vi "Agilent SNA Measure.vi"(5 "Miscellaneous Parameters":T1, 7 "Agilent SNA & SWP":T6, 8 "error in (no error)":errorcluster, 9 "SP Stimulus":T2={"Use Instrument Settings"=FALSE, "Blank Frequencies"=FALSE, "Sweep Type"=enum."Linear", "Sweep"={"Fstart"=500.0, "Fstop"=1500.0, "Units"=enum."MHz", "Points"=201}, "Power (dBm)"=999.0, "IFBW (Hz)"=-1.0, "Sweep Time (s)"=-1.0, "Calibration"={"State"=FALSE, "String"=""}} {"Sweep Time (s)" format="%.3g"}, 10 "Parameters to Measure":T7[](array[typedef]) {"Channel" min=1 max=99 step=1; "Parameter"."Stimulus Port" min=1 step=1; "Parameter"."Response Port" min=1 step=1}, 11 "VISA Resource Names":T5) -> (0 "error out":errorcluster, 1 "S Parameters":cluster{"f0":dbl, "df":dbl, cdb[][]}, 2 "Parameters to Measure":T7[](array[typedef]) {"Channel" min=1 max=99 step=1; "Parameter"."Stimulus Port" min=1 step=1; "Parameter"."Response Port" min=1 step=1}, 3 "dup VISA Resource Names":T5)   [LabVIEW 2011]
uses:
  tests/S Parameter/TypeDefs/SP Parameter to Measure.ctl
  tests/S Parameter/TypeDefs/SP Parameter.ctl
  tests/S Parameter/TypeDefs/SP Calibration State.ctl
  tests/S Parameter/TypeDefs/SP Measurement Format.ctl
  TypeDefs/Agilent SNA VISA.ctl
  TypeDefs/Agilent SNA Instrument Info.ctl
  tests/S Parameter/TypeDefs/SP Stimulus Parameters.ctl
  tests/S Parameter/TypeDefs/SP Frequency Units.ctl
  tests/S Parameter/TypeDefs/SP Miscellaneous Parameters.ctl
  TypeDefs/Agilent SNA Message Mode.ctl
  TypeDefs/Agilent SNA Measurement.ctl
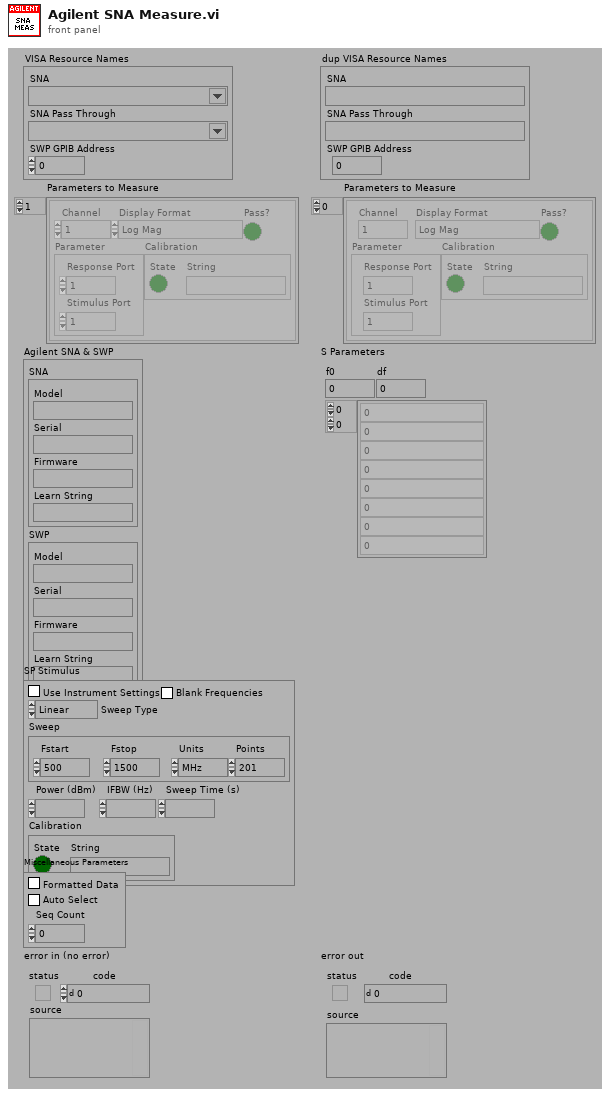
[diagram p1: front panel]
types:
  T1 = typedef "SP Miscellaneous Parameters.ctl" = cluster{"Formatted Data":bool, "Auto Select":bool, "Seq Count":u32}
  T2 = typedef "SP Stimulus Parameters.ctl" = cluster{"Use Instrument Settings":bool, "Blank Frequencies":bool, "Sweep Type":enum32{"Linear", "Logarithmic", "List", "Power", "CW"}, "Sweep":cluster{"Fstart":dbl, "Fstop":dbl, "Units":T3, "Points":i32}, "Power (dBm)":dbl, "IFBW (Hz)":dbl, "Sweep Time (s)":dbl, "Calibration":T4}
  T3 = typedef "SP Frequency Units.ctl" = enum16{"Hz", "kHz", "MHz", "GHz", "Points"}
  T4 = typedef "SP Calibration State.ctl" = cluster{"State":bool, "String":string}
  T5 = typedef "Agilent SNA VISA.ctl" = cluster{"SNA":refnum<visa-resource-name>, "SNA Pass Through":refnum<visa-resource-name>, "SWP GPIB Address":i32}
  T6 = typedef "Agilent SNA Instrument Info.ctl" = cluster{"SNA":cluster{"Model":string, "Serial":string, "Firmware":string, "Learn String":string}, "SWP":cluster{"Model":string, "Serial":string, "Firmware":string, "Learn String":string}}
  T7 = typedef "SP Parameter to Measure.ctl" = cluster{"Channel":i8, "Parameter":T8, "Calibration":T4, "Display Format":T9, "Pass?":bool}
  T8 = typedef "SP Parameter.ctl" = cluster{"Stimulus Port":i8, "Response Port":i8}
  T9 = typedef "SP Measurement Format.ctl" = enum32{"Log Mag", "Phase", "Delay", "Smith (R+jX)", "Polar (Re/Im)", "Linear Mag", "SWR", "Real", "Imaginary", "Smith (Lin/Phase)", "Smith (Log/Phase)", "Smith (Real/Imag)", "Smith (G+jB)", "Polar (Lin/Phase)", "Polar (Log/Phase)", "Expanded Phase", "Positive Phase", "Inverted Smith", "Unwrapped Phase", "Power Out", "Power In", "Linear Mag/Phase", "Log Mag/Phase", "Real/Imaginary"}
  T10 = typedef "Agilent SNA Message Mode.ctl" = enum16{"On", "Off"}
  T11 = typedef "Agilent SNA Model.ctl" = enum16{"Not Supported", "8757X"}
  T12 = typedef "Agilent SNA Measurement.ctl" = enum32{"SXX", "A", "B", "C", "R", "A/B", "A/C", "A/R", "B/A", "B/C", "B/R", "C/A", "C/B", "C/R", "R/A", "R/B", "R/C", "Analog In - Aux In"}
  T13 = typedef "Agilent SNA Measurements.ctl" = cluster{"Channel":i8, "Traces":cluster{"Trace":i8, "Parameter":T8}[]}
  T14 = typedef "Agilent SNA Trigger Mode.ctl" = enum16{"Continuous", "Hold", "Single"}
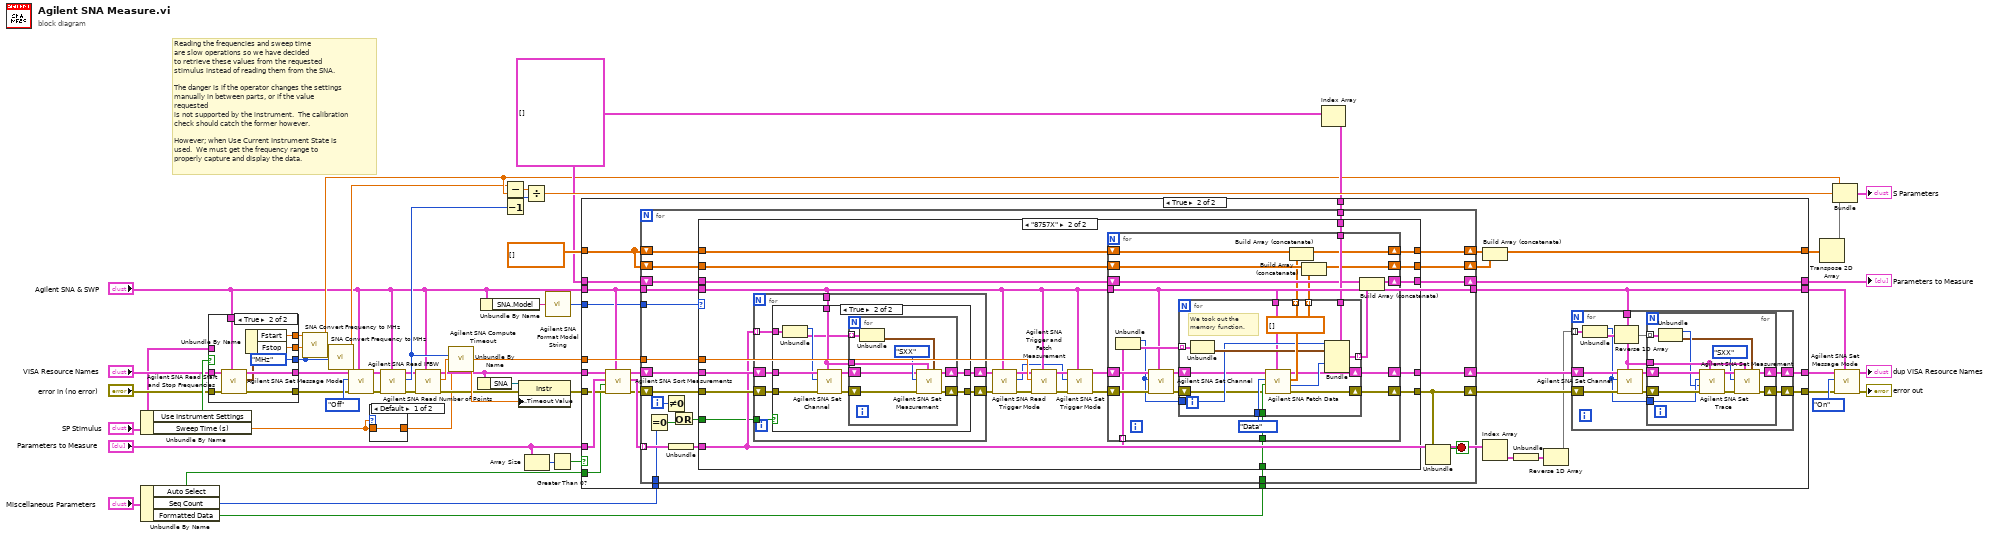
[diagram p0: block diagram]
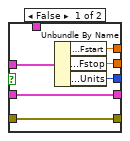
[diagram p2: hidden frame]
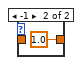
[diagram p3: hidden frame]
diagram:
  w33 = T7[] [] ("Parameters to Measure")
  # "Reading the frequencies and sweep time\nare slow operations so we have decided\nto retrieve these values from the requested\nstimulus instead of reading them from the SNA.\n\nThe danger is if the operator changes the settings\nmanually in between parts, or if the value requested\nis not supported by the instrument.  The calibration\ncheck should catch the former however.\n\nHowever; when Use Current Instrument State is\nused.  We must get the frequency range to\nproperly capture and display the data."
  n1 = Unbundle By Name("SP Stimulus") -> ("Use Instrument Settings"=w10:bool, "Sweep Time (s)"=w26:dbl)
  n2 = Unbundle By Name("Miscellaneous Parameters") -> ("Auto Select"=w34:bool, "Seq Count"=w28:u32, "Formatted Data"=w29:bool)
  n3 = case shown="True" w10 {
    tunnel: "VISA Resource Names" -> [w56 w63]
    tunnel: "error in (no error)" -> [w57 w66]
    tunnel: [w57 w65] -> w7
    tunnel: [w56 w64] -> w6
    tunnel: "Agilent SNA & SWP" -> [_ w62]
    tunnel: "SP Stimulus" -> [w55 _]
    tunnel: [w54 w60] -> w3
    tunnel: [w53 w59] -> w2
    tunnel: [w52 SP_Frequency_Units."MHz" ("Units")] -> w1
    frame False {
      n4 = Unbundle By Name(w55) -> ("Sweep.Fstart"=w54:dbl, "Sweep.Fstop"=w53:dbl, "Sweep.Units"=w52:T3)
    }
    frame True {
      n5 = call "Agilent SNA Read Start and Stop Frequencies.vi"("Agilent SNA & SWP"=w62, "error in (no error)"=w66, "VISA Resource Names"=w63) -> ("error out"=w65:errorcluster, "Start/Stop Freqs, MHz"=w61:cluster{"Fstart":dbl, "Fstop":dbl}, "dup VISA Resource Names"=w64:T5)  [unwired: 2 in, 4 out]
      n6 = Unbundle By Name(w61) -> ("Fstart"=w60:dbl, "Fstop"=w59:dbl)
    }
  }
  n7 = call "SNA Convert Frequency to MHz.vi"("Units"=w1, "Frequency"=w3) -> ("Converted Frequency"=w21:dbl)  [unwired: 9 out]
  n8 = call "SNA Convert Frequency to MHz.vi"("Units"=w1, "Frequency"=w2) -> ("Converted Frequency"=w20:dbl)  [unwired: 9 out]
  n9 = call "Agilent SNA Set Message Mode.vi"("Agilent SNA & SWP"="Agilent SNA & SWP", "error in (no error)"=w7, "Message Mode"=Agilent_SNA_Message_Mode."Off", "VISA Resource Names"=w6) -> ("error out"=w16:errorcluster, "dup VISA Resource Names"=w17:T5)  [unwired: 6 out]
  n10 = case shown="Default" w26 {
    tunnel: w26 -> [w67 _]
    tunnel: [w67 1.0 ("Sweep Time (s)")] -> w22
    frame Default {
    }
    frame -1 {
    }
  }
  n11 = call "Agilent SNA Read Number of Points.vi"("Agilent SNA & SWP"="Agilent SNA & SWP", "error in (no error)"=w16, "VISA Resource Names"=w17) -> ("error out"=w38:errorcluster, "Number Points"=w40:i32, "dup VISA Resource Names"=w39:T5)  [unwired: 1 in, 5 out]
  n12 = call "Agilent SNA Read IFBW.vi"("Agilent SNA & SWP"="Agilent SNA & SWP", "error in (no error)"=w38, "VISA Resource Names"=w39) -> ("error out"=w23:errorcluster, "IFBW, Hz"=w25:dbl, "dup VISA Resource Name"=w24:T5)  [unwired: 1 in, 5 out]
  n13 = call "Agilent SNA Compute Timeout.vi"("Points"=w40, "IFBW (Hz)"=w25, "Sweep Time (s)"=w22) -> ("Timeout (ms)"=w41:dbl)  [unwired: 1 in, 11 out]
  n14 = Unbundle By Name(w24) -> ("SNA"=w27:refnum<visa-resource-name>)
  n15 = Unbundle By Name("Agilent SNA & SWP") -> ("SNA.Model"=w31:string)
  n16 = Subtract(x=w20, y=w21) -> (x-y=w50:dbl)
  n17 = Decrement(x=w40) -> (x-1=w49:i32)
  n18 = property class="Instr"(reference=w27, error in=w23, "General Settings:Timeout Value"=w41) -> (error out=w43:errorcluster)  [unwired: 1 out]
  n19 = Divide(x=w50, y=w49) -> (x/y=w47:dbl)
  n20 = Array Size(array="Parameters to Measure") -> (size(s)=w45:i32)
  n21 = call "Agilent SNA Format Model String.vi"("Model String"=w31) -> ("Model"=w30:T11)
  n22 = Greater Than 0?(x=w45) -> (x > 0?=w44:bool)
  n23 = Index Array(array=w33) -> (element=w32:T7)  [unwired: 1 in]
  n24 = case shown="True" w44 {
    tunnel: [w73 w95] -> w13
    tunnel: w24 -> [w71 w81]
    tunnel: "Parameters to Measure" -> [_ w100]
    tunnel: [w72 w88] -> w51
    tunnel: "Agilent SNA & SWP" -> [w69 w79]
    tunnel: w43 -> [w73 w84]
    tunnel: cdb[][] [] -> [w72 w91]
    tunnel: [w71 w94] -> w12
    tunnel: w41 -> [_ w92]
    tunnel: w29 -> [_ w87]
    tunnel: [w70 w86] -> w36
    tunnel: w33 -> [w70 w85]
    tunnel: w34 -> [_ w80]
    tunnel: w32 -> [_ w78]
    tunnel: w30 -> [_ w76]
    tunnel: w28 -> [_ w75]
    tunnel: [w69 w74] -> w11
    frame False {
    }
    frame True {
      n25 = call "Agilent SNA Sort Measurements.vi"("Agilent SNA & SWP"=w79, "error in (no error)"=w84, "Auto Select"=w80, "Parameters to Measure"=w100, "VISA Resource Names"=w81) -> ("error out"=w83:errorcluster, "Sorted Measurements"=w99:cluster{"Measurements":T13[]}[], "dup VISA Resource Names"=w82:T5)  [unwired: 4 out]
      n26 = for {
        shift-right: [w120] -> w96
        shift-left: w83 -> [w122]
        tunnel: w99 -> [w107] mode=indexing
        tunnel: w79 -> [w109]
        shift-right: [w110] -> w89
        shift-left: w91 -> [w115]
        shift-right: [w121] -> w97
        shift-left: w82 -> [w123]
        tunnel: [w109] -> w74
        tunnel: w92 -> [w119]
        shift-right: [w111] -> w90
        shift-left: w91 -> [w114]
        tunnel: w87 -> [w118]
        shift-right: [w112] -> w86
        shift-left: w85 -> [w113]
        tunnel: w78 -> [w116]
        tunnel: w76 -> [w108]
        tunnel: w75 -> [w102]
        i -> [w103]
        stop <- w117 stop-if-true
        n27 = Equal To 0?(x=w102) -> (x = 0?=w105:bool)
        n28 = Not Equal To 0?(x=w103) -> (x != 0?=w104:bool)
        n29 = Unbundle(w107) -> ("Measurements"=w106:T13[])
        n30 = Or(x=w104, y=w105) -> (x .or. y?=w101:bool)
        n31 = case shown="\"8757X\"" w108 {
          tunnel: w123 -> [w127 w153]
          tunnel: w122 -> [w128 w152]
          tunnel: [w127 w151] -> w121
          tunnel: [w128 w150] -> w120
          tunnel: w119 -> [_ w149]
          tunnel: w118 -> [_ w148]
          tunnel: w116 -> [_ w147]
          tunnel: w115 -> [w125 w146]
          tunnel: w114 -> [w126 w145]
          tunnel: w113 -> [w124 w144]
          tunnel: [w124 w143] -> w112
          tunnel: [w126 w142] -> w111
          tunnel: [w125 w141] -> w110
          tunnel: w109 -> [_ w131]
          tunnel: w106 -> [_ w140]
          tunnel: w101 -> [_ w129]
          frame "Not Supported" {
          }
          frame "8757X" {
            n32 = for {
              tunnel: w131 -> [w192]
              tunnel: w140 -> [w195] mode=indexing
              shift-right: [w193] -> w138
              shift-left: w152 -> [w196]
              shift-right: [w194] -> w139
              shift-left: w153 -> [w197]
              tunnel: w129 -> [w191]
              n33 = case shown="True" w191 {
                tunnel: w197 -> [w199 w209]
                tunnel: w196 -> [w198 w208]
                tunnel: w195 -> [_ w207]
                tunnel: [w199 w206] -> w194
                tunnel: [w198 w205] -> w193
                tunnel: w192 -> [_ w204]
                frame False {
                  # "Save time because we know that the previous\nrun set these measurements back to the first\nparameters.  The cannot be skipped if it is the\nsecond measurement in a run though or if it is\nthe first time through."
                }
                frame True {
                  n34 = Unbundle(w207) -> ("Channel"=w203:i8, "Traces"=w202:cluster{"Trace":i8, "Parameter":T8}[])
                  n35 = call "Agilent SNA Set Channel.vi"("Agilent SNA & SWP"=w204, "error in (no error)"=w208, "Channel"=w203, "VISA Resource Names"=w209) -> ("error out"=w201:errorcluster, "dup VISA Resource Names"=w200:T5)  [unwired: 6 out]
                  n36 = for {
                    tunnel: w204 -> [w215]
                    tunnel: w202 -> [w214] mode=indexing
                    shift-right: [w217] -> w206
                    shift-left: w200 -> [w211]
                    shift-right: [w216] -> w205
                    shift-left: w201 -> [w210]
                    n37 = Unbundle(w214) -> ("Parameter"=w212:T8)  [unwired: 1 out]
                    n38 = call "Agilent SNA Set Measurement.vi"("Parameter"=w212, "Agilent SNA & SWP"=w215, "error in (no error)"=w210, "Measurement (SXX)"=Agilent_SNA_Measurement."SXX" ("Measurement (S11 - A/R)"), "VISA Resource Names"=w211) -> ("error out"=w216:errorcluster, "dup VISA Resource Names"=w217:T5)  [unwired: 2 in, 3 out]
                  }
                }
              }
            }
            n39 = call "Agilent SNA Read Trigger Mode.vi"("Agilent SNA & SWP"=w131, "error in (no error)"=w138, "VISA Resource Names"=w139) -> ("error out"=w137:errorcluster, "Trigger Mode"=w130:T14, "dup VISA Resource Names"=w136:T5)  [unwired: 1 in, 5 out]
            n40 = call "Agilent SNA Trigger and Fetch Measurement.vi"("Agilent SNA & SWP"=w131, "error in (no error)"=w137, "Timout, ms (10000)"=w149, "VISA Resource Names"=w136) -> ("error out"=w135:errorcluster, "dup VISA Resource Names"=w134:T5)  [unwired: 2 in, 4 out]
            n41 = call "Agilent SNA Set Trigger Mode.vi"("Agilent SNA & SWP"=w131, "error in (no error)"=w135, "Trigger Mode"=w130, "VISA Resource Names"=w134) -> ("error out"=w132:errorcluster, "dup VISA Resource Names"=w133:T5)  [unwired: 1 in, 5 out]
            n42 = for {
              shift-right: [w155] -> w150
              shift-left: w132 -> [w175]
              tunnel: w140 -> [w168] mode=indexing
              shift-right: [w156] -> w151
              shift-left: w133 -> [w174]
              tunnel: w148 -> [w172]
              tunnel: w147 -> [w169]
              tunnel: w131 -> [w154]
              shift-right: [w162] -> w141
              shift-left: w146 -> [w165]
              shift-right: [w160] -> w143
              shift-left: w144 -> [w163]
              shift-right: [w161] -> w142
              shift-left: w145 -> [w164]
              n43 = Unbundle(w168) -> ("Channel"=w166:i8, "Traces"=w167:cluster{"Trace":i8, "Parameter":T8}[])
              n44 = call "Agilent SNA Set Channel.vi"("Agilent SNA & SWP"=w154, "error in (no error)"=w175, "Channel"=w166, "VISA Resource Names"=w174) -> ("error out"=w170:errorcluster, "dup VISA Resource Names"=w171:T5)  [unwired: 6 out]
              n45 = for {
                tunnel: [w190] -> w157 mode=indexing
                tunnel: [cdb[] [] ("Data (real+imag)")] -> w158 mode=indexing
                tunnel: enum16{"Data", "Memory"}."Data" ("Data to Read (Data)") -> [w189]
                tunnel: w172 -> [w188]
                tunnel: [w186] -> w159 mode=indexing
                tunnel: w166 -> [w182]
                tunnel: w169 -> [w185]
                shift-right: [w180] -> w156
                shift-left: w171 -> [w178]
                shift-right: [w179] -> w155
                shift-left: w170 -> [w177]
                tunnel: w167 -> [w184] mode=indexing
                tunnel: w154 -> [w176]
                # "We took out the\nmemory function."
                n46 = Unbundle(w184) -> ("Parameter"=w183:T8)  [unwired: 1 out]
                n47 = call "Agilent SNA Fetch Data.vi"("Agilent SNA & SWP"=w176, "error in (no error)"=w177, "Formatted Data?"=w188, "Data to Read (Data)"=w189, "VISA Resource Names"=w178) -> ("error out"=w179:errorcluster, "Display Format"=w187:T9, "Data (real+imag)"=w190:cdb[], "dup VISA Resource Names"=w180:T5)  [unwired: 2 in, 1 out]
                n48 = Bundle(cluster=w185, "Channel"=w182, "Parameter"=w183, "Display Format"=w187) -> (w186:T7)  [unwired: 2 out]
              }
              n49 = Build Array (concatenate)(w165, w157) -> (w162:cdb[][])
              n50 = Build Array (concatenate)(w164, w158) -> (w161:cdb[][])
              n51 = Build Array (concatenate)(w163, w159) -> (w160:T7[])
            }
          }
        }
        n52 = Unbundle(w120) -> ("status"=w117:bool)  [unwired: 2 out]
      }
      n53 = Build Array (concatenate)(w89, w90) -> (w88:cdb[][])
      n54 = Index Array(array=w99) -> (element=w98:cluster{"Measurements":T13[]})  [unwired: 1 in]
      n55 = Unbundle(w98) -> ("Measurements"=w77:T13[])
      n56 = Reverse 1D Array(array=w77) -> (reversed array=w93:T13[])
      n57 = for {
        tunnel: w74 -> [w223]
        tunnel: w93 -> [w226] mode=indexing
        shift-right: [w220] -> w95
        shift-left: w96 -> [w227]
        shift-right: [w219] -> w94
        shift-left: w97 -> [w228]
        n58 = Unbundle(w226) -> ("Channel"=w221:i8, "Traces"=w222:cluster{"Trace":i8, "Parameter":T8}[])
        n59 = Reverse 1D Array(array=w222) -> (reversed array=w218:cluster{"Trace":i8, "Parameter":T8}[])
        n60 = call "Agilent SNA Set Channel.vi"("Agilent SNA & SWP"=w223, "error in (no error)"=w227, "Channel"=w221, "VISA Resource Names"=w228) -> ("error out"=w225:errorcluster, "dup VISA Resource Names"=w224:T5)  [unwired: 6 out]
        n61 = for {
          tunnel: w223 -> [w234]
          tunnel: w221 -> [w233]
          tunnel: w218 -> [w232] mode=indexing
          shift-right: [w240] -> w219
          shift-left: w224 -> [w235]
          shift-right: [w239] -> w220
          shift-left: w225 -> [w238]
          n62 = Unbundle(w232) -> ("Trace"=w231:i8, "Parameter"=w230:T8)
          n63 = call "Agilent SNA Set Trace.vi"("Agilent SNA & SWP"=w234, "error in (no error)"=w238, "Trace"=w231, "Channel"=w233, "VISA Resource Names"=w235) -> ("error out"=w237:errorcluster, "dup VISA Resource Names"=w236:T5)  [unwired: 5 out]
          n64 = call "Agilent SNA Set Measurement.vi"("Parameter"=w230, "Agilent SNA & SWP"=w234, "error in (no error)"=w237, "Measurement (SXX)"=Agilent_SNA_Measurement."SXX" ("Measurement (S11 - A/R)"), "VISA Resource Names"=w236) -> ("error out"=w239:errorcluster, "dup VISA Resource Names"=w240:T5)  [unwired: 2 in, 3 out]
        }
      }
    }
  }
  "Parameters to Measure" <- w36
  n65 = Transpose 2D Array(2D array=w51) -> (transposed array=w46:cdb[][])
  n66 = Bundle("Converted Frequency"=w21, w47, w46) -> (→"S Parameters":cluster{"Converted Frequency":dbl, dbl, cdb[][]})  [unwired: 1 out]
  n67 = call "Agilent SNA Set Message Mode.vi"("Agilent SNA & SWP"=w11, "error in (no error)"=w13, "Message Mode"=Agilent_SNA_Message_Mode."On", "VISA Resource Names"=w12) -> ("error out"=→"error out":errorcluster, "dup VISA Resource Names"=→"dup VISA Resource Names":T5)  [unwired: 6 out]
